vi "Build table array.vi"(11 "Table details":T1(array[cluster])) -> (3 "Column details":string[][](array[string]))   [LabVIEW 2015]
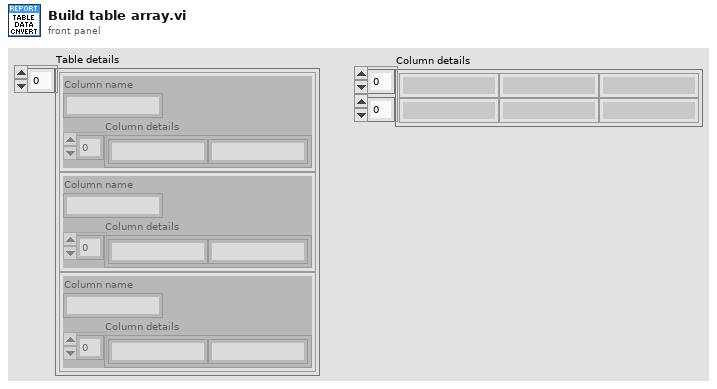
[diagram p1: front panel]
types:
  T1 = cluster{"Column name":string, "Column details":string[]}[]
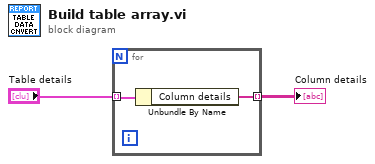
[diagram p0: block diagram]
diagram:
  n1 = for {
    tunnel: "Table details" -> [w4] mode=indexing
    tunnel: [w3] -> w1 mode=indexing
    n2 = Unbundle By Name(w4) -> ("Column details"=w3:string[])
  }
  "Column details" <- w1
